vi "Calculate Desired States.vi"(8 "error in (no error)":errorcluster, 10 "Vessel In":refnum<class "Vessel.lvclass">, 11 "Joystick Guidance in":refnum<class "Joystick Guidance.lvclass">) -> (0 "error out":errorcluster, 2 "Vessel Out":refnum<class "Vessel.lvclass">, 3 "Joystick Guidance out":refnum<class "Joystick Guidance.lvclass">)   [LabVIEW 2014, in "Guidance Library.lvlib" / "Joystick Guidance.lvclass"]
uses:
  Joystick Guidance.lvclass
  ROV/Vessel.lvclass
  Joystick Guidance.lvclass/Joystick Guidance.ctl
  <vilib>/Analysis/baseanly.llb/A x Vector.vi
  Library/Kinematics/J_euler.vi
  Library/Helping Routines/get_set_point_vec (SubVI).vi
  Library/Helping Routines/get_set_point (SubVI).vi
  Reference Models/Reference Model Joystick.vi
  Library/Integrator/Integrator trapez vector.vi
  Supervisor/Supervisor.lvclass
  <vilib>/Analysis/NI_AALBase.lvlib
panel:
  out "sway":cluster{"Numeric":dbl, "Numeric":dbl}(graph)
  out "Surge":cluster{"Numeric":dbl, "Numeric":dbl}(graph)
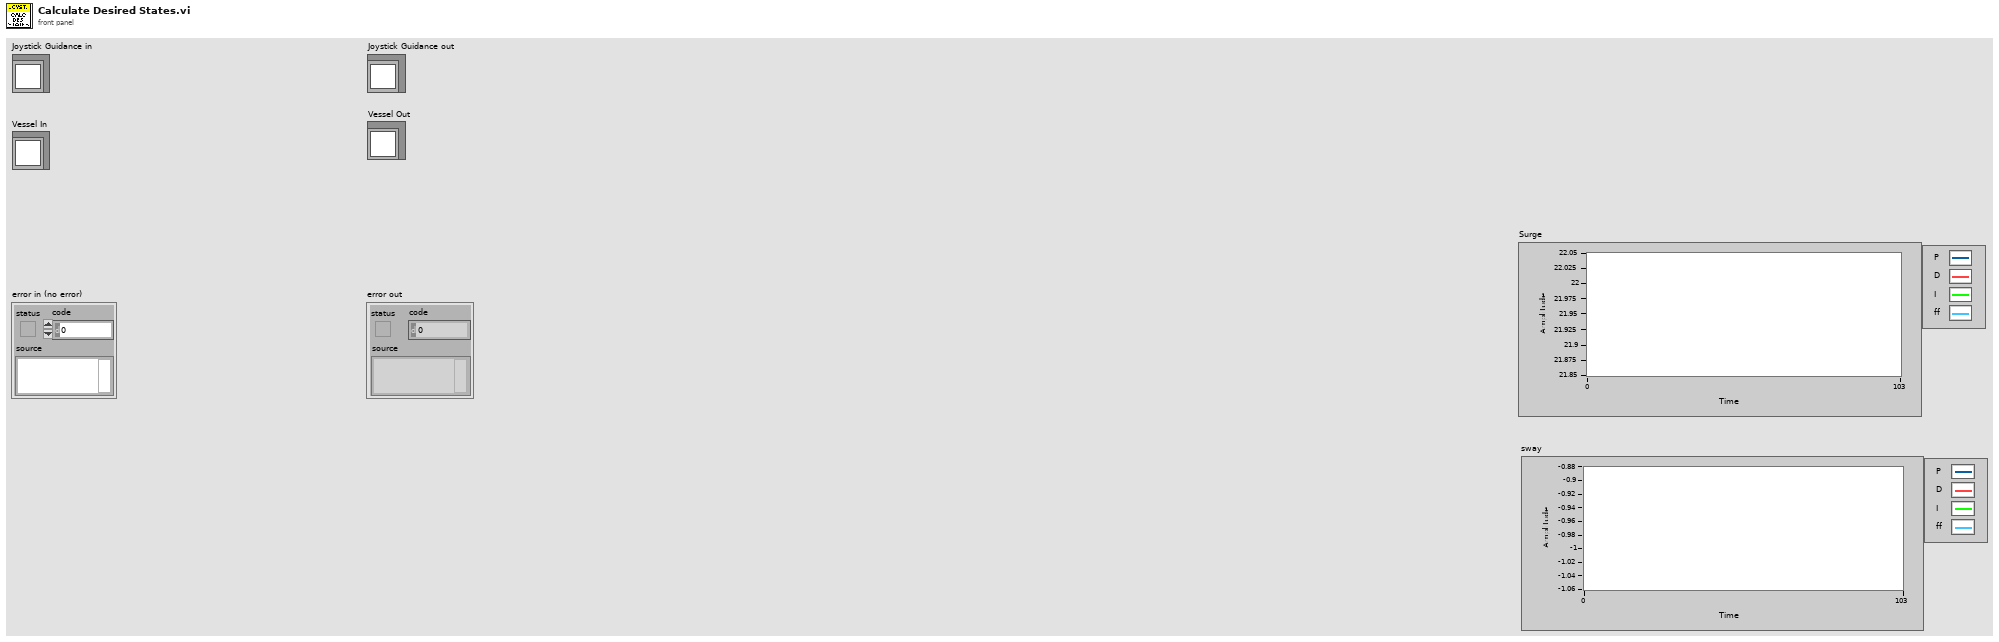
[diagram p1: front panel]
types:
  T1 = cluster{"Axis Translation":cluster{"X-Axis":dbl, "Y-Axis":dbl, "Z-Axis":dbl}, "Axis Rotation":cluster{"X-Axis":dbl, "Y-Axis":dbl, "Z-Axis":dbl}}
  T2 = cluster{"Button 1":bool, "Button 2":bool, "Button 3":bool, "Button 4":bool, "Button 5":bool, "Button 6":bool, "Button 7":bool, "Button 8":bool, "Button 9":bool, "Button 10":bool, "Button 11":bool, "Button 12":bool, "POV Direction":i32}
  T3 = cluster{"Measured":cluster{"Eta":dbl[], "Nu":dbl[], "Eta Dot":dbl[], "Nu Dot":dbl[]}, "Estimated":cluster{"Eta":dbl[], "Nu":dbl[], "Eta Dot":dbl[], "Nu Dot":dbl[]}, "Desired":cluster{"Eta":dbl[], "Nu":dbl[], "Eta Dot":dbl[], "Nu Dot":dbl[]}, "Previous Desired":cluster{"Eta":dbl[], "Nu":dbl[], "Eta Dot":dbl[], "Nu Dot":dbl[]}, "tau":dbl[], "Altitude":cluster{"Measured":dbl, "Estimated":dbl, "Desired":dbl, "Previous Desired":dbl, "Approximated":dbl, "grad F":dbl[]}, "rpm":dbl[], "Attitude":cluster{"Theta Measured":dbl[], "Theta Estimated":dbl[], "Omega Measured":dbl[], "Omega Estimated":dbl[], "Gyro Bias":dbl[]}}
  T4 = typedef "NI_Matrix.lvlib/RealMatrix.ctl" = dbl[][]
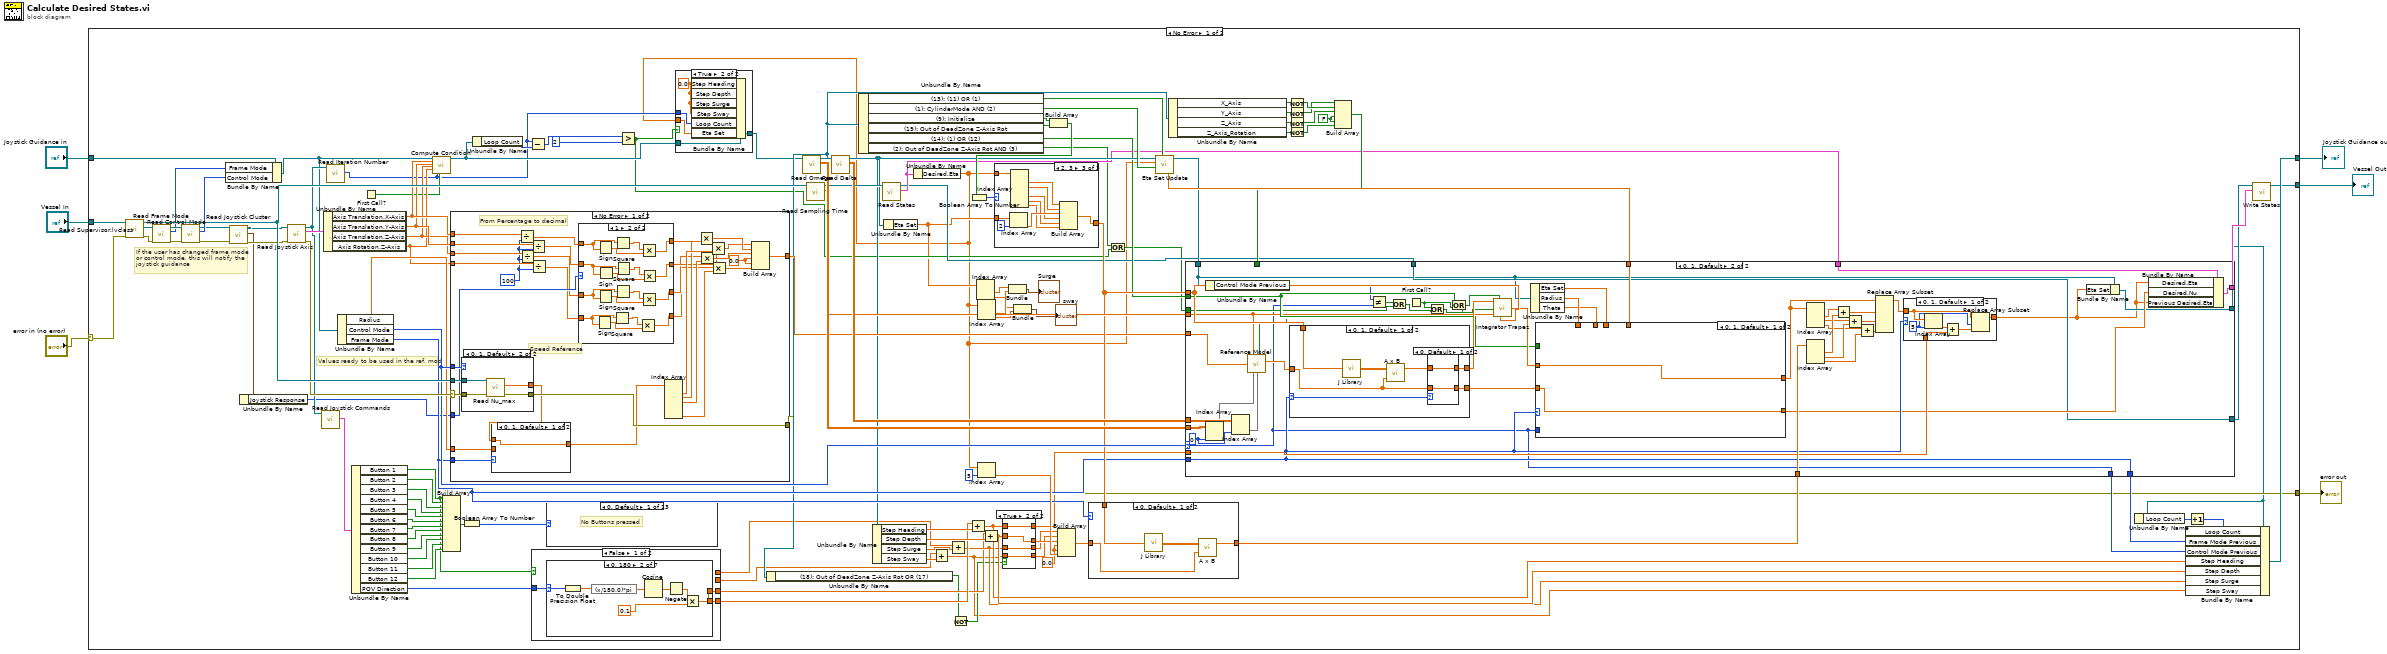
[diagram p0: block diagram]
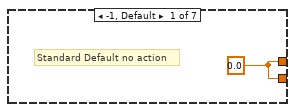
[diagram p2: hidden frame]
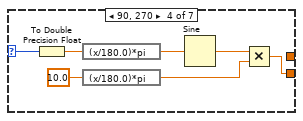
[diagram p4: hidden frame]
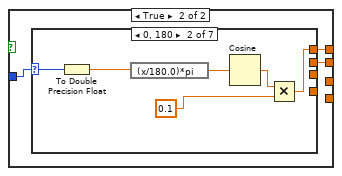
[diagram p8: hidden frame]
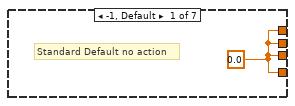
[diagram p9: hidden frame]
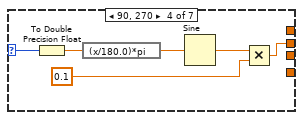
[diagram p11: hidden frame]
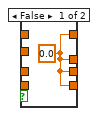
[diagram p16: hidden frame]
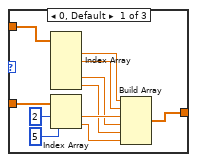
[diagram p18: hidden frame]
diagram:
  n1 = case shown="No Error" "error in (no error)" {
    selector: "error in (no error)" -> [w127 w444]
    tunnel: "Vessel In" -> [w129 w445]
    tunnel: "Joystick Guidance in" -> [w56 w446]
    tunnel: [w95 w446] -> w3
    tunnel: [w58 w445] -> w2
    tunnel: [w59 w444] -> w1
    frame No Error {
      w62 = FALSE
      w98 = 0.0 ("element")
      # "If the user has changed frame mode\nor control mode, this will notify the\njoystick guidance"
      # "Values ready to be used in the ref. mod"
      n2 = call "Read Supervisor.lvclass.vi"("error in (no error)"=w127, "Vessel in"=w129) -> ("error out"=w50:errorcluster, "Supervisor.lvclass"=w54:refnum<class "Supervisor.lvclass">, "Vessel out"=w126:refnum<class "Vessel.lvclass">)  [unwired: 7 in]
      n3 = call-dynamic "Read Frame Mode.vi"("error in (no error)"=w50, "Supervisor in"=w54) -> ("error out"=w49:errorcluster, "Frame Mode Previous"=w51:u16, "Supervisor out"=w53:refnum<class "Supervisor.lvclass">)  [unwired: 7 in]
      n4 = call-dynamic "Read Control Mode.vi"("error in (no error)"=w49, "Supervisor in"=w53) -> ("error out"=w20:errorcluster, "Control Mode"=w52:u16, "Supervisor out"=w22:refnum<class "Supervisor.lvclass">)  [unwired: 7 in]
      n5 = Bundle By Name(cluster=w56, "Frame Mode"=w51, "Control Mode"=w52) -> (w55:refnum<class "Joystick Guidance.lvclass">)
      n6 = call-dynamic "Read Joystick Cluster.vi"("error in (no error)"=w20, "Supervisor in"=w22) -> ("error out"=w19:errorcluster, "Joystick Cluster"=w18:cluster{"Joystick Response":u16}, "Supervisor out"=w21:refnum<class "Supervisor.lvclass">)  [unwired: 7 in]
      n7 = Unbundle By Name(w18) -> ("Joystick Response"=w17:u16)
      n8 = call-dynamic "Read Joystick Axis.vi"("error in (no error)"=w19, "Supervisor in"=w21) -> ("error out"=w122:errorcluster, "Joystick Axis"=w128:T1, "Supervisor out"=w82:refnum<class "Supervisor.lvclass">)  [unwired: 7 in]
      n9 = call-dynamic "Read Joystick Commands.vi"("Supervisor in"=w82) -> ("Joystick Commands"=w121:T2)  [unwired: 8 in, 2 out]
      n10 = Unbundle By Name(w128) -> ("Axis Translation.X-Axis"=w86:dbl, "Axis Translation.Y-Axis"=w85:dbl, "Axis Translation.Z-Axis"=w84:dbl, "Axis Rotation.Z-Axis"=w83:dbl)
      n11 = call-dynamic "Read Iteration Number.vi"("Supervisor in"=w82) -> ("Iteration Number"=w39:i32)  [unwired: 8 in, 2 out]
      n12 = Unbundle By Name(w55) -> ("Radius"=w93:dbl, "Control Mode"=w94:u16, "Frame Mode"=w90:u16)
      n13 = Unbundle By Name(w121) -> ("Button 1"=w26:bool, "Button 2"=w119:bool, "Button 3"=w118:bool, "Button 4"=w117:bool, "Button 5"=w116:bool, "Button 6"=w115:bool, "Button 7"=w114:bool, "Button 8"=w113:bool, "Button 9"=w112:bool, "Button 10"=w111:bool, "Button 11"=w110:bool, "Button 12"=w109:bool, "POV Direction"=w120:i32)
      n14 = First Call?() -> (First Call?: T/F=w81:bool)
      n15 = call "Compute Condition.vi"("Joystick Guidance in"=w55, "X-Axis"=w86, "Y-Axis"=w85, "Z-Axis"=w84, "Z-Axis Rotation"=w83, "Loop Nr"=w39, "First"=w81) -> ("Joystick Guidance out"=w44:refnum<class "Joystick Guidance.lvclass">)  [unwired: 11 in, 1 out]
      n16 = Build Array(w26, w119, w118, w117, w116, w115, w114, w113, w112, w111, w110, w109) -> (w107:bool[])
      n17 = case shown="No Error" w122 {
        selector: w122 -> [w389 w443]
        tunnel: w86 -> [w410 _]
        tunnel: w85 -> [w409 _]
        tunnel: w84 -> [w408 _]
        tunnel: w83 -> [w407 _]
        tunnel: [w398 _] -> w78
        tunnel: w126 -> [w390 _]
        tunnel: [w397 w443] -> w59
        tunnel: w94 -> [w395 _]
        tunnel: w90 -> [w394 _]
        tunnel: w93 -> [w391 _]
        tunnel: w17 -> [w387 _]
        frame No Error {
          w396 = 0.0
          w406 = 100
          # "From Percentage to decimal"
          # "Speed Reference"
          n18 = case shown="0, 1, Default" w395 {
            tunnel: [w438 w442] -> w393
            tunnel: w390 -> [w437 w441]
            tunnel: w389 -> [w436 w440]
            tunnel: [w435 w439] -> w397
            frame 2, 3 {
              n19 = call "Read Max Thrust.vi"("error in (no error)"=w436, "Vessel in"=w437) -> ("error out"=w435:errorcluster, "Max Thrust"=w438:dbl[])  [unwired: 7 in, 1 out]
            }
            frame 0, 1, Default {
              n20 = call "Read Nu_max.vi"("error in (no error)"=w440, "Vessel in"=w441) -> ("error out"=w439:errorcluster, "Nu_max"=w442:dbl[])  [unwired: 7 in, 1 out]
            }
          }
          n21 = case shown="0, 1, Default" w394 {
            tunnel: w393 -> [w431 w434]
            tunnel: [w431 w433] -> w392
            tunnel: w391 -> [_ w432]
            frame 0, 1, Default {
            }
            frame 2 {
              n22 = call "Cylinder Kinematics Modification.vi"("Radius"=w432, "Max Velocity"=w434) -> ("Max Velocity Modified"=w433:dbl[])
            }
          }
          n23 = Divide(x=w410, y=w406) -> (x/y=w386:dbl)
          n24 = Divide(x=w408, y=w406) -> (x/y=w382:dbl)
          n25 = Divide(x=w409, y=w406) -> (x/y=w384:dbl)
          n26 = Divide(x=w407, y=w406) -> (x/y=w380:dbl)
          n27 = case shown="1" w387 {
            tunnel: w386 -> [w414 w420]
            tunnel: [w414 w419] -> w385
            tunnel: w384 -> [w413 w418]
            tunnel: [w413 w417] -> w383
            tunnel: w382 -> [w412 w416]
            tunnel: [w412 w415] -> w381
            tunnel: w380 -> [w411 w430]
            tunnel: [w411 w427] -> w379
            frame 0, Default {
            }
            frame 1 {
              n28 = Sign(1:w430) -> (0:w429:dbl)
              n29 = Sign(1:w420) -> (0:w421:dbl)
              n30 = Sign(1:w416) -> (0:w425:dbl)
              n31 = Sign(1:w418) -> (0:w424:dbl)
              n32 = Square(x=w430) -> (x^2=w428:dbl)
              n33 = Square(x=w420) -> (x^2=w422:dbl)
              n34 = Square(x=w416) -> (x^2=w426:dbl)
              n35 = Square(x=w418) -> (x^2=w423:dbl)
              n36 = Multiply(x=w428, y=w429) -> (x*y=w427:dbl)
              n37 = Multiply(x=w422, y=w421) -> (x*y=w419:dbl)
              n38 = Multiply(x=w426, y=w425) -> (x*y=w415:dbl)
              n39 = Multiply(x=w423, y=w424) -> (x*y=w417:dbl)
            }
          }
          n40 = Index Array(array=w392) -> (element #1=w405:dbl, element #2=w404:dbl, element #3=w403:dbl, element #6=w388:dbl)  [unwired: 6 in, 2 out]
          n41 = Multiply(x=w385, y=w404) -> (x*y=w402:dbl)
          n42 = Multiply(x=w381, y=w403) -> (x*y=w400:dbl)
          n43 = Multiply(x=w383, y=w405) -> (x*y=w401:dbl)
          n44 = Multiply(x=w379, y=w388) -> (x*y=w399:dbl)
          n45 = Build Array(w401, w402, w400, w396, w396, w399) -> (w398:dbl[])
        }
        frame Error {
        }
      }
      n46 = Boolean Array To Number(Boolean array=w107) -> (number=w108:u32)
      n47 = Unbundle By Name(w44) -> ("Loop Count"=w40:i32)
      n48 = Subtract(x=w39, y=w40) -> (x-y=w46:i32)
      n49 = case shown="False" w26 {
        tunnel: w120 -> [w132 w148]
        tunnel: [w131 _] -> w33
        tunnel: [w130 _] -> w29
        tunnel: [_ w150] -> w24
        tunnel: [_ w149] -> w25
        frame False {
          n50 = case shown="0, 180" w132 {
            selector: w132 -> [_ w140 _ w146 _ _ _]
            tunnel: [w133 w136 _ _ _ _ _] -> w130
            tunnel: [w133 _ _ w141 _ _ _] -> w131
            frame -1, Default {
              w133 = 0.0
              # "Standard Default no action"
            }
            frame 0, 180 {
              n51 = To Double Precision Float(number=w140) -> (double precision float=w139:dbl)
              n52 = expression code="(x/180.0)*pi" ("degrees to radians")(w139) -> (w138:dbl)
              n53 = Cosine(x=w138) -> (cos(x)=w135:dbl)
              n54 = Negate(x=w135) -> (-x=w134:dbl)
              n55 = Multiply(x=w134, y=0.1) -> (x*y=w136:dbl)
            }
            frame 45 {
            }
            frame 90, 270 {
              n56 = To Double Precision Float(number=w146) -> (double precision float=w145:dbl)
              n57 = expression code="(x/180.0)*pi" ("degrees to radians")(w145) -> (w144:dbl)
              n58 = expression code="(x/180.0)*pi" ("degrees to radians")(10.0) -> (w142:dbl)
              n59 = Sine(x=w144) -> (sin(x)=w143:dbl)
              n60 = Multiply(x=w143, y=w142) -> (x*y=w141:dbl)
            }
            frame 135 {
            }
            frame 225 {
            }
            frame 315 {
            }
          }
        }
        frame True {
          n61 = case shown="0, 180" w148 {
            selector: w148 -> [_ w157 _ w163 _ _ _]
            tunnel: [w151 _ _ _ _ _ _] -> _
            tunnel: [w151 _ _ _ _ _ _] -> _
            tunnel: [w151 _ _ w158 _ _ _] -> w150
            tunnel: [w151 w152 _ _ _ _ _] -> w149
            frame -1, Default {
              w151 = 0.0
              # "Standard Default no action"
            }
            frame 0, 180 {
              n62 = To Double Precision Float(number=w157) -> (double precision float=w156:dbl)
              n63 = expression code="(x/180.0)*pi" ("degrees to radians")(w156) -> (w155:dbl)
              n64 = Cosine(x=w155) -> (cos(x)=w154:dbl)
              n65 = Multiply(x=w154, y=0.1) -> (x*y=w152:dbl)
            }
            frame 45 {
            }
            frame 90, 270 {
              n66 = To Double Precision Float(number=w163) -> (double precision float=w162:dbl)
              n67 = expression code="(x/180.0)*pi" ("degrees to radians")(w162) -> (w161:dbl)
              n68 = Sine(x=w161) -> (sin(x)=w160:dbl)
              n69 = Multiply(x=w160, y=0.1) -> (x*y=w158:dbl)
            }
            frame 135 {
            }
            frame 225 {
            }
            frame 315 {
            }
          }
        }
      }
      n70 = case shown="0, Default" w108 {
        frame 0, Default {
          # "No Buttons pressed"
        }
        frame 1 {
          # "Button 1 Pressed"
        }
        frame 2 {
          # "Button 2 Pressed"
        }
        frame 4 {
          # "Button 3 pressed"
        }
        frame 8 {
          # "Button 4 Pressed"
        }
        frame 16 {
          # "Button 5 pressed"
        }
        frame 32 {
          # "Button 6 Pressed"
        }
        frame 64 {
          # "Button 7 Pressed"
        }
        frame 128 {
          # "Button 8 Pressed"
        }
        frame 256 {
          # "Button 9 Pressed"
        }
        frame 512 {
          # "Button 10 Pressed"
        }
        frame 1024 {
          # "Button 11 Pressed"
        }
        frame 2048 {
          # "Button 12 Pressed"
        }
      }
      n71 = Greater?(x=w46, y=2) -> (0:w41:bool)
      n72 = call-dynamic "Read Sampling Time.vi"("Vessel in"=w126) -> ("Sampling Time"=w105:dbl, "Vessel out"=w92:refnum<class "Vessel.lvclass">)  [unwired: 8 in, 1 out]
      n73 = call-dynamic "Read States.vi"("Vessel in"=w92) -> ("States"=w60:T3, "Vessel out"=w48:refnum<class "Vessel.lvclass">)  [unwired: 8 in, 1 out]
      n74 = Unbundle By Name(w60) -> ("Desired.Eta"=w11:dbl[])
      n75 = case shown="True" w41 {
        tunnel: w44 -> [w164 w169]
        tunnel: [w164 w168] -> w43
        tunnel: w11 -> [_ w167]
        tunnel: w39 -> [_ w166]
        frame False {
        }
        frame True {
          w165 = 0.0
          n76 = Bundle By Name(cluster=w169, "Step Heading"=w165, "Step Depth"=w165, "Step Surge"=w165, "Step Sway"=w165, "Loop Count"=w166, "Eta Set"=w167) -> (w168:refnum<class "Joystick Guidance.lvclass">)
        }
      }
      n77 = call-dynamic "Read Omega.vi"("Guidance in"=w43) -> ("Omega"=w123:T4, "Guidance out"=w125:refnum<class "Joystick Guidance.lvclass">)  [unwired: 8 in, 1 out]
      n78 = call-dynamic "Read Delta.vi"("Guidance in"=w125) -> ("Delta"=w124:T4, "Guidance out"=w68:refnum<class "Joystick Guidance.lvclass">)  [unwired: 8 in, 1 out]
      n79 = Unbundle By Name(w68) -> ("(18): Out of DeadZone Z-Axis Rot OR (17)"=w28:bool)
      n80 = Unbundle By Name(w68) -> ("(13): (11) OR (1)"=w79:bool, "(1): CylinderMode AND (2)"=w80:bool, "(9): Initialize"=w77:bool, "(19): Out of DeadZone Z-Axis Rot"=w76:bool, "(14): (1) OR (12)"=w67:bool, "(2): Out of DeadZone Z-Axis Rot AND (3)"=w16:bool)
      n81 = Unbundle By Name(w68) -> ("Step Heading"=w104:dbl, "Step Depth"=w103:dbl, "Step Surge"=w101:dbl, "Step Sway"=w102:dbl)
      n82 = Unbundle By Name(w68) -> ("Eta Set"=w13:dbl[])
      n83 = Add(x=w24, y=w102) -> (x+y=w23:dbl)
      n84 = Add(x=w25, y=w101) -> (x+y=w32:dbl)
      n85 = Not(x=w28) -> (.not. x?=w27:bool)
      n86 = Add(x=w33, y=w104) -> (x+y=w34:dbl)
      n87 = Index Array(array=w13) -> (element #1=w12:dbl, element #2=w8:dbl)  [unwired: 2 in]
      n88 = Index Array(array=w11) -> (element #1=w10:dbl, element #2=w7:dbl)  [unwired: 2 in]
      n89 = Index Array(array=w11, index=5) -> (element=w99:dbl)
      n90 = Add(x=w29, y=w103) -> (x+y=w35:dbl)
      n91 = case shown="True" w27 {
        tunnel: [w170 w174] -> w15
        tunnel: [w170 w173] -> w69
        tunnel: [w170 w172] -> w31
        tunnel: [w170 w171] -> w30
        tunnel: w34 -> [_ w174]
        tunnel: w35 -> [_ w173]
        tunnel: w32 -> [_ w172]
        tunnel: w23 -> [_ w171]
        frame False {
          w170 = 0.0
        }
        frame True {
        }
      }
      n92 = Bundle("Numeric"=w12, "Numeric"=w10) -> (→"Surge":cluster{"Numeric":dbl, "Numeric":dbl})  [unwired: 1 in]
      n93 = Bundle("Numeric"=w8, "Numeric"=w7) -> (→"sway":cluster{"Numeric":dbl, "Numeric":dbl})  [unwired: 1 in]
      n94 = Build Array(w77, w76) -> (w75:bool[])
      n95 = Boolean Array To Number(Boolean array=w75) -> (number=w106:u32)
      n96 = case shown="2, 3" w106 {
        tunnel: [w185 w191 w200] -> w91
        tunnel: w11 -> [w184 w191 w201]
        tunnel: w13 -> [w183 _ w197]
        frame 0, Default {
          n97 = Index Array(array=w184) -> (element #1=w186:dbl, element #2=w187:dbl, element #4=w180:dbl, element #5=w181:dbl)  [unwired: 5 in, 1 out]
          n98 = Index Array(array=w183, index #1=2 ("index"), index #2=5 ("index")) -> (element #1=w188:dbl, element #2=w182:dbl)
          n99 = Build Array(w186, w187, w188, w180, w181, w182) -> (w185:dbl[])
        }
        frame 1 {
        }
        frame 2, 3 {
          n100 = Index Array(array=w197, index=2) -> (element=w195:dbl)
          n101 = Index Array(array=w201) -> (element #1=w199:dbl, element #2=w198:dbl, element #4=w192:dbl, element #5=w193:dbl, element #6=w194:dbl)  [unwired: 6 in, 1 out]
          n102 = Build Array(w199, w198, w195, w192, w193, w194) -> (w200:dbl[])
        }
      }
      n103 = Build Array(w31, w30, w69, w98, w98, w99) -> (w97:dbl[])
      n104 = case shown="0, Default" w90 {
        tunnel: w97 -> [w177 w179]
        tunnel: [w178 w179] -> w96
        tunnel: w91 -> [w176 _]
        frame 0, Default {
          n105 = call-poly "J Library.vi"("eta"=w176) -> ("J"=w175:T4)
          n106 = call-poly <vilib>:"A x B.vi"("Vector"=w177, "A"=w175) -> ("A x Vector"=w178:dbl[])  [unwired: 1 out]
        }
        frame 1, 2 {
        }
      }
      n107 = Or(x=w16, y=w41) -> (x .or. y?=w42:bool)
      n108 = call "Eta Set Update.vi"("CylinderMode"=w79, "Condition"=w80, "Eta"=w11, "Joystick Guidance in"=w68) -> ("Joystick Guidance out"=w74:refnum<class "Joystick Guidance.lvclass">, "Heading Calculated"=w89:dbl)  [unwired: 3 in, 3 out]
      n109 = Unbundle By Name(w68) -> ("X_Axis"=w73:bool, "Y_Axis"=w72:bool, "Z_Axis"=w71:bool, "Z_Axis_Rotation"=w70:bool)
      n110 = Not(x=w73) -> (.not. x?=w66:bool)
      n111 = Not(x=w72) -> (.not. x?=w65:bool)
      n112 = Not(x=w71) -> (.not. x?=w64:bool)
      n113 = Not(x=w70) -> (.not. x?=w63:bool)
      n114 = Build Array(w65, w66, w64, w62, w62, w63) -> (w61:bool[])
      n115 = case shown="0, 1, Default" w94 {
        selector: w94 -> [w268 w280]
        tunnel: w78 -> [w266 w293]
        tunnel: w91 -> [_ w309]
        tunnel: w105 -> [_ w292]
        tunnel: w124 -> [_ w323]
        tunnel: w123 -> [_ w322]
        tunnel: w74 -> [w270 w283]
        tunnel: [w258 w295] -> w38
        tunnel: w96 -> [_ w321]
        tunnel: w15 -> [_ w310]
        tunnel: w90 -> [w269 w300]
        tunnel: w89 -> [_ w302]
        tunnel: [w269 w300] -> w88
        tunnel: [w268 w280] -> w87
        tunnel: w67 -> [_ w294]
        tunnel: w42 -> [_ w285]
        tunnel: w61 -> [w264 _]
        tunnel: w60 -> [w257 w298]
        tunnel: [w267 w296] -> w57
        tunnel: w48 -> [w261 w288]
        tunnel: [w260 w288] -> w47
        frame 2, 3 {
          w234 = dbl[] [0.0, 0.0, 0.0, 0.0, 0.0, 0.0] ("Desired.Nu")
          w238 = FALSE ("element")
          w240 = 0.0
          n116 = Bundle By Name(cluster=w270, "Thrust"=w266) -> (w259:refnum<class "Joystick Guidance.lvclass">)
          n117 = call "Read Supervisor.lvclass.vi"("Vessel in"=w261) -> ("error out"=w262:errorcluster, "Supervisor.lvclass"=w265:refnum<class "Supervisor.lvclass">, "Vessel out"=w263:refnum<class "Vessel.lvclass">)  [unwired: 8 in]
          n118 = call-dynamic "Write Joystick Thruster Select.vi"("error in (no error)"=w262, "Joystick Thruster Select"=w264, "Supervisor in"=w265) -> ("error out"=w216:errorcluster, "Supervisor out"=w217:refnum<class "Supervisor.lvclass">)  [unwired: 7 in]
          n119 = call-dynamic "Read Iteration Number.vi"("error in (no error)"=w216, "Supervisor in"=w217) -> ("error out"=w215:errorcluster, "Supervisor out"=w214:refnum<class "Supervisor.lvclass">)  [unwired: 7 in, 1 out]
          n120 = call-dynamic "Read Joystick setpoint array.vi"("error in (no error)"=w215, "Supervisor in"=w214) -> ("error out"=w224:errorcluster, "Joystick setpoint array"=w223:bool[], "Supervisor out"=w225:refnum<class "Supervisor.lvclass">)  [unwired: 7 in]
          n121 = Index Array(array=w223, index=2) -> ()  [unwired: 1 out]
          n122 = call-dynamic "Read Use Altitude Guidance.vi"("error in (no error)"=w224, "Supervisor in"=w225) -> ("error out"=w227:errorcluster, "Use Altitude Guidance"=w218:bool, "Supervisor out"=w226:refnum<class "Supervisor.lvclass">)  [unwired: 7 in]
          n123 = Not(x=w218) -> (.not. x?=w219:bool)
          n124 = feedback #1() -> (w221:bool)  [unwired: 1 in]
          n125 = Not Equal?(x=w218, y=w221) -> (x != y?=w220:bool)
          n126 = feedback-in #1(w218) -> ()
          n127 = And(x=w219, y=w220) -> (x .and. y?=w213:bool)
          n128 = feedback #2(10) -> (w212:i32)
          n129 = case shown="True" w213 {
            tunnel: [w276 0] -> w210
            tunnel: w212 -> [w275 _]
            frame False {
              n130 = Add(x=w275, y=1) -> (x+y=w276:i32)
            }
            frame True {
            }
          }
          n131 = feedback-in #2(w210) -> ()
          n132 = case shown="1, Default" w210 {
            tunnel: [TRUE ("element") FALSE ("element") TRUE ("element")] -> w209
            frame 0 {
            }
            frame 1, Default {
            }
            frame 2 {
            }
          }
          n133 = call-dynamic "Read Joystick Commands.vi"("error in (no error)"=w227, "Supervisor in"=w226) -> ("error out"=w236:errorcluster, "Joystick Commands"=w256:T2, "Supervisor out"=w237:refnum<class "Supervisor.lvclass">)  [unwired: 7 in]
          n134 = Unbundle By Name(w257) -> ("Estimated.Eta"=w255:dbl[])
          n135 = Unbundle By Name(w256) -> ("Button 5"=w245:bool, "Button 2"=w208:bool, "Button 3"=w247:bool)
          n136 = Or(x=w209, y=w208) -> (x .or. y?=w207:bool)
          n137 = Index Array(array=w255, index #1=0 ("index"), index #2=1 ("index"), index #3=2 ("index"), index #4=5 ("index")) -> (element #1=w250:dbl, element #2=w249:dbl, element #3=w246:dbl, element #4=w244:dbl)
          n138 = Build Array(w250, w249) -> (w248:dbl[])
          n139 = call-poly "Get Set Point (SubVI).vi"("Set point in"=w248, "auto set  in"=w247) -> ("auto set"=w202:bool, "Set point"=w243:dbl[])
          n140 = call-poly "Get Set Point (SubVI).vi"("set point in"=w246, "auto set  in"=w207) -> ("auto set"=w229:bool, "set point"=w242:dbl)
          n141 = call-poly "Get Set Point (SubVI).vi"("set point in"=w244, "auto set  in"=w245) -> ("auto set"=w228:bool, "set point"=w241:dbl)
          n142 = Build Array (concatenate)(w243, w242, w240, w240, w241) -> (w239:dbl[])
          n143 = Build Array(w202, w202, w229, w238, w238, w228) -> (w235:bool[])
          n144 = call-dynamic "Write Joystick setpoint array.vi"("error in (no error)"=w236, "Joystick setpoint array"=w235, "Supervisor in"=w237) -> ("error out"=w204:errorcluster, "Supervisor out"=w206:refnum<class "Supervisor.lvclass">)  [unwired: 7 in]
          n145 = call-dynamic "Write Auto pos.vi"("error in (no error)"=w204, "Auto pos"=w202, "Supervisor in"=w206) -> ("error out"=w203:errorcluster, "Supervisor out"=w205:refnum<class "Supervisor.lvclass">)  [unwired: 7 in]
          n146 = Bundle By Name(cluster=w257, "tau"=w266, "Desired.Eta"=w239, "Desired.Nu"=w234, "Desired.Eta Dot"=w234) -> (w267:T3)
          n147 = call-dynamic "Write Auto Depth.vi"("error in (no error)"=w203, "Auto Depth"=w229, "Supervisor in"=w205) -> ("error out"=w232:errorcluster, "Supervisor out"=w233:refnum<class "Supervisor.lvclass">)  [unwired: 7 in]
          n148 = Bundle By Name(cluster=w259, "Eta Set"=w239) -> (w258:refnum<class "Joystick Guidance.lvclass">)
          n149 = call-dynamic "Write Auto Heading.vi"("error in (no error)"=w232, "Auto Heading"=w228, "Supervisor in"=w233) -> ("error out"=w231:errorcluster, "Supervisor out"=w230:refnum<class "Supervisor.lvclass">)  [unwired: 7 in]
          n150 = call "Write Supervisor.lvclass.vi"("error in (no error)"=w231, "Supervisor.lvclass"=w230, "Vessel in"=w263) -> ("Vessel out"=w260:refnum<class "Vessel.lvclass">)  [unwired: 7 in, 1 out]
        }
        frame 0, 1, Default {
          w299 = 0
          n151 = Unbundle By Name(w283) -> ("Control Mode Previous"=w281:u16)
          n152 = Index Array(array=w322, index (col)=w299) -> (element=w290:dbl[])  [unwired: 1 in]
          n153 = Index Array(array=w323, index (col)=w299) -> (element=w289:dbl[])  [unwired: 1 in]
          n154 = Not Equal?(x=w281, y=w280) -> (x != y?=w282:bool)
          n155 = Or(x=w282, y=w285) -> (x .or. y?=w284:bool)
          n156 = First Call?() -> (First Call?: T/F=w287:bool)
          n157 = Or(x=w287, y=w284) -> (x .or. y?=w286:bool)
          n158 = Or(x=w294, y=w287) -> (x .or. y?=w278:bool)
          n159 = call-poly "Reference Model.vi"("dt"=w292, "Reset"=w278, "Reference Joystick"=w293, "Omega"=w290, "Delta"=w289) -> ("nu_desired"=w291:dbl[])  [unwired: 9 in, 1 out]
          n160 = case shown="0, 1, Default" w300 {
            selector: w300 -> [w366 _]
            tunnel: w291 -> [w364 w371]
            tunnel: w309 -> [w361 _]
            tunnel: [w363 w371] -> w308
            tunnel: [w362 w371] -> w304
            frame 0, 1, Default {
              n161 = call-poly "J Library.vi"("eta"=w361) -> ("J"=w360:T4)
              n162 = call-poly <vilib>:"A x B.vi"("Vector"=w364, "A"=w360) -> ("A x Vector"=w365:dbl[])  [unwired: 1 out]
              n163 = case shown="0, Default" w366 {
                tunnel: w365 -> [w368 w370]
                tunnel: w364 -> [w367 w369]
                tunnel: [w368 w369] -> w363
                tunnel: [w367 w370] -> w362
                frame 0, Default {
                }
                frame 1 {
                }
              }
            }
            frame 2 {
            }
          }
          n164 = call-poly "Integrator Trapez.vi"("IC"=w309, "Reset"=w278, "dt"=w292, "Initialize"=w286, "Input"=w308) -> ("Output"=w307:dbl[])  [unwired: 1 in]
          n165 = Unbundle By Name(w283) -> ("Eta Set"=w303:dbl[], "Radius"=w305:dbl, "Theta"=w301:dbl)
          n166 = case shown="0, 1, Default" w300 {
            tunnel: w307 -> [w325 w352]
            tunnel: [w325 w337] -> w306
            tunnel: w305 -> [_ w351]
            tunnel: w280 -> [_ w334]
            tunnel: w304 -> [w324 w332]
            tunnel: [w324 w333] -> w297
            tunnel: w301 -> [_ w331]
            tunnel: w303 -> [_ w330]
            tunnel: w302 -> [_ w327]
            tunnel: w294 -> [_ w326]
            frame 0, 1, Default {
            }
            frame 2 {
              w339 = 0.0
              n167 = Index Array(array=w352) -> (element #1=w350:dbl, element #2=w347:dbl, element #3=w344:dbl)  [unwired: 3 in]
              n168 = Subtract(x=w351, y=w350) -> (x-y=w349:dbl)
              n169 = Subtract(x=w331, y=w347) -> (x-y=w348:dbl)
              n170 = Index Array(array=w330) -> (element #1=w329:dbl, element #2=w328:dbl)  [unwired: 2 in]
              n171 = Polar To Re/Im(2:w348, 3:w349) -> (0:w343:dbl, 1:w342:dbl)
              n172 = Add(x=w329, y=w342) -> (x+y=w346:dbl)
              n173 = Inverse Tangent (2 Input)(1:w342, 2:w343) -> (0:w341:dbl)
              n174 = Add(x=w328, y=w343) -> (x+y=w345:dbl)
              n175 = Add(x=w341, y=3.141592653589793) -> (x+y=w336:dbl)
              n176 = Build Array(w346, w345, w344, w339, w339, w336) -> (w338:dbl[])
              n177 = Select(t=w336, s=w326, f=w327) -> (s? t:f=w335:dbl)
              n178 = case shown="0, 2, 3, Default" w334 {
                tunnel: [dbl[] [0.0, 0.0, 0.0, 0.0, 0.0, 0.0] w354] -> w333
                tunnel: w332 -> [_ w354]
                frame 0, 2, 3, Default {
                }
                frame 1 {
                }
              }
              n179 = case shown="1, 2" w334 {
                tunnel: w338 -> [w355 w359]
                tunnel: [w355 w358] -> w337
                tunnel: w335 -> [_ w357]
                frame 0, Default {
                }
                frame 1, 2 {
                  n180 = Replace Array Subset(array=w359, new element=w357, index=5) -> (w358:dbl[])
                }
              }
            }
          }
          n181 = Index Array(array=w306) -> (element #1=w314:dbl, element #2=w313:dbl, element #3=w312:dbl)  [unwired: 3 in]
          n182 = Index Array(array=w321) -> (element #1=w317:dbl, element #2=w316:dbl, element #3=w315:dbl)  [unwired: 3 in]
          n183 = Add(x=w314, y=w317) -> (x+y=w320:dbl)
          n184 = Add(x=w313, y=w316) -> (x+y=w319:dbl)
          n185 = Add(x=w312, y=w315) -> (x+y=w318:dbl)
          n186 = Replace Array Subset(array=w306, new element #1=w320, new element #2=w319, new element #3=w318) -> (w311:dbl[])  [unwired: 3 in]
          n187 = case shown="0, 1, Default" w300 {
            tunnel: w311 -> [w374 w378]
            tunnel: w310 -> [w376 _]
            tunnel: [w372 w378] -> w279
            frame 0, 1, Default {
              w373 = 5 ("index")
              n188 = Index Array(array=w374, index=w373) -> (element=w377:dbl)
              n189 = Add(x=w377, y=w376) -> (x+y=w375:dbl)
              n190 = Replace Array Subset(array=w374, new element=w375, index=w373) -> (w372:dbl[])
            }
            frame 2 {
            }
          }
          n191 = Bundle By Name(cluster=w283, "Eta Set"=w279) -> (w295:refnum<class "Joystick Guidance.lvclass">)
          n192 = Bundle By Name(cluster=w298, "Desired.Eta"=w279, "Desired.Nu"=w297, "Previous Desired.Eta"=w279) -> (w296:T3)
        }
      }
      n193 = Unbundle By Name(w38) -> ("Loop Count"=w37:i32)
      n194 = Increment(x=w37) -> (x+1=w36:i32)
      n195 = Bundle By Name(cluster=w38, "Loop Count"=w36, "Frame Mode Previous"=w88, "Control Mode Previous"=w87, "Step Heading"=w34, "Step Depth"=w35, "Step Surge"=w32, "Step Sway"=w23) -> (w95:refnum<class "Joystick Guidance.lvclass">)
      n196 = call-dynamic "Write States.vi"("States"=w57, "Vessel in"=w47) -> ("Vessel out"=w58:refnum<class "Vessel.lvclass">)  [unwired: 8 in, 1 out]
    }
    frame Error {
    }
  }
  "error out" <- w1
  "Joystick Guidance out" <- w3
  "Vessel Out" <- w2
